vi "COP FSM.vi"   [LabVIEW 2009]
uses:
  COP Support Files/COP FSM States.ctl
  Support Files/JUDP Write Queue Element.ctl
  <vilib>/Platform/TimedLoop/XDataNode/XDataNode.xnode
  <vilib>/Platform/TimedLoop/XDataNode/loadlvalarms.vi
  <vilib>/Platform/TimedLoop/XDataNode/timing_clust.ctl
  <vilib>/Platform/TimedLoop/XDataNode/nitl_modes.ctl
  <vilib>/Platform/TimedLoop/XDataNode/wakeup.ctl
  <vilib>/Platform/TimedLoop/XDataNode/XDNodeRunTimeDep.lvlib
types:
  T1 = typedef "JUDP Write Queue Element.ctl" = cluster{"Encoded JAUS Message":string, "Destination ID":u32}
  T2 = typedef "COP FSM States.ctl" = enum16{"QueryStatus", "rQueryIdentification", "sReportIdentification", "sQueryServices", "rReportServices", "sQueryControl", "rReportControl", "sRequestControl", "rConfirmControl", "sResume", "sStandby", "sShutdown", "sQueryVelocityState", "sQueryLocalPose", "rSendWaypoints", "rExecuteWaypoints"}
  T3 = typedef "XDNodeRunTimeDep.lvlib/timing_clust.ctl" = cluster{"Expected End [f-1]":u64, "Actual End [f-1]":u64, "Finished Late? [f-1]":bool, "Expected End [i-1]":u64, "Actual End [i-1]":u64, "Finished Late? [i-1]":bool, "Expected Start [i]":u64, "Actual Start [i]":u64, "Expected Start [f]":u64, "Actual Start [f]":u64, "Source Name":string, "Structure Name":string, "Period":i64, "Deadline":i64, "Offset":i64, "Start":i64, "Priority":i32, "Timeout":i32, "Mode":T4, "Wakeup Reason":T5, "Error":errorcluster, "Source Type":string, "Secondary Source Type":string, "Global End Time":u64, "Global Start Time":u64, "Frame Duration":u64, "Iteration Duration":u64, "Assigned CPU":i32, "I/O Scan Engine Mode":u32}
  T4 = typedef "XDNodeRunTimeDep.lvlib/nitl_modes.ctl" = enum32{"No Change", "Process missed periods, maintain original phase", "Discard missed periods, maintain original phase", "Process missed periods, ignore original phase", "Discard missed periods, ignore original phase"}
  T5 = typedef "XDNodeRunTimeDep.lvlib/wakeup.ctl" = enum32{"Normal", "Aborted", "Asynchronous wakeup", "Timing source error", "Timed loop error", "Timeout"}
  T6 = typedef "Address.ctl" = cluster{"Subsystem Id":u16, "Node Id":u8, "Component Id":u8}
  T7 = typedef "RequestIDRec.ctl" = cluster{"RequestId":u8, "Element List":T8[]}
  T8 = typedef "ElementRec.ctl" = cluster{"ElementUID":u16, " PreviousUID":u16, " NextUID":u16, "LocalWaypointRec":T9}
  T9 = typedef "LocalWaypointRec.ctl" = cluster{"Presence Vector":u8, " X":dbl, " Y":dbl, " Z":dbl, "Roll":dbl, "Pitch":dbl, "Yaw":dbl, "Waypoint Tolerance":dbl, "Path Tolerance":dbl, "Is Active?":bool}
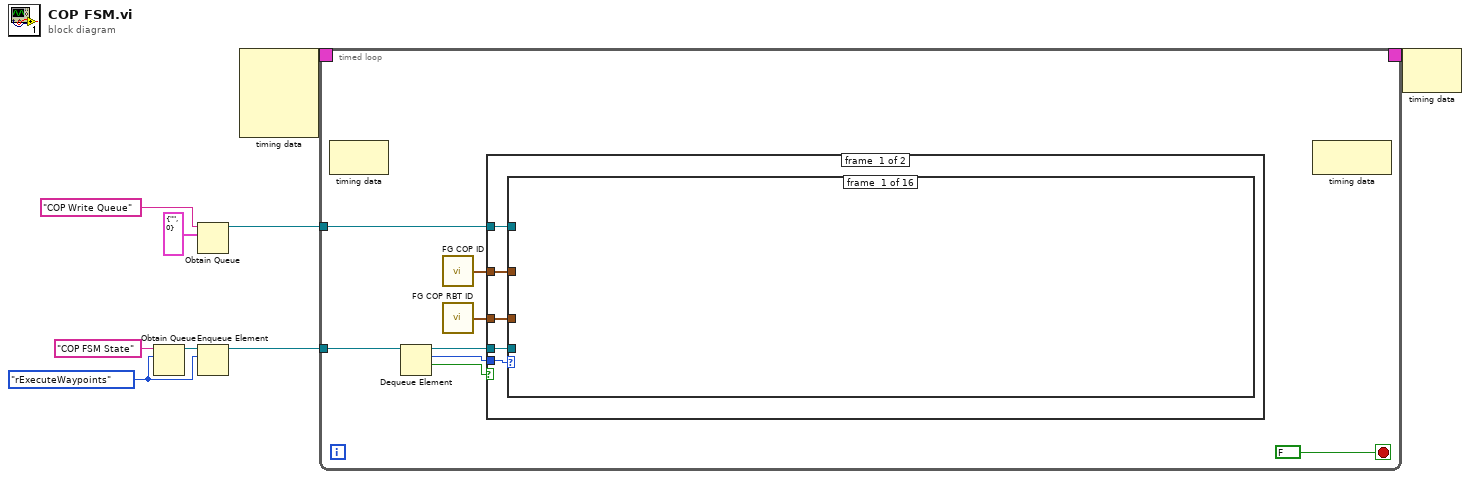
[diagram p0: block diagram]
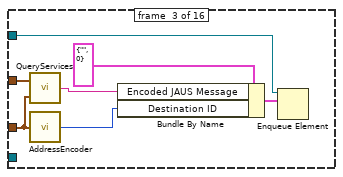
[diagram p3: hidden frame]
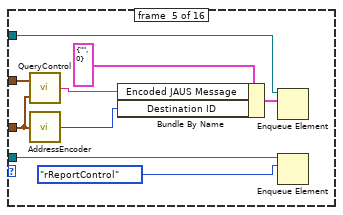
[diagram p5: hidden frame]
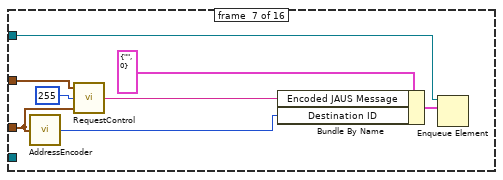
[diagram p7: hidden frame]
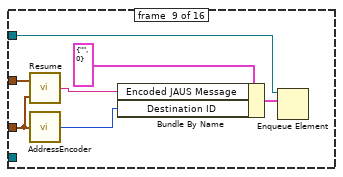
[diagram p9: hidden frame]
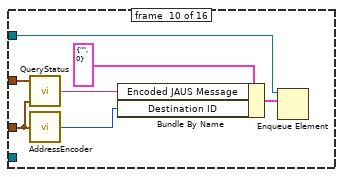
[diagram p10: hidden frame]
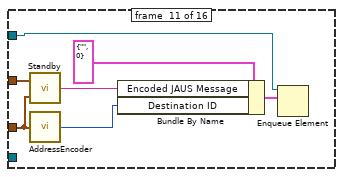
[diagram p11: hidden frame]
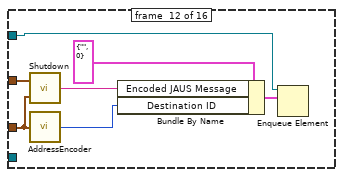
[diagram p12: hidden frame]
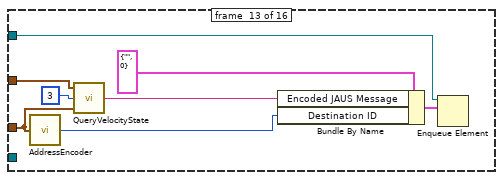
[diagram p13: hidden frame]
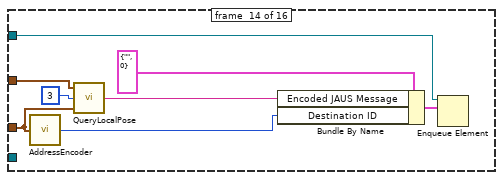
[diagram p14: hidden frame]
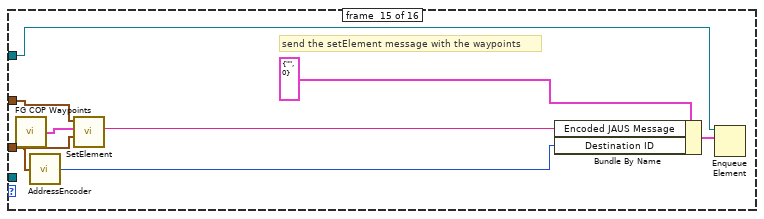
[diagram p15: hidden frame]
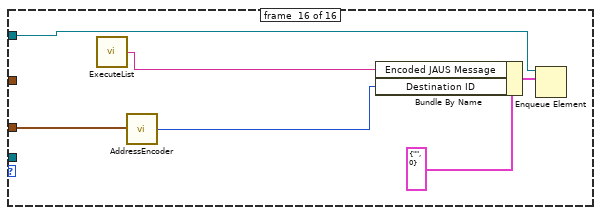
[diagram p16: hidden frame]
diagram:
  w6 = COP_FSM_States."rExecuteWaypoints" ("COP FSM States")
  n1 = Obtain Queue(name (unnamed)="COP FSM State", element data type=w6) -> (queue out=w8:refnum<queue>)  [unwired: 3 in, 2 out]
  n2 = Obtain Queue(name (unnamed)="COP Write Queue", element data type=T1 {"Encoded JAUS Message"="", "Destination ID"=0} ("Cluster")) -> (queue out=w3:refnum<queue>)  [unwired: 3 in, 2 out]
  n3 = Enqueue Element(queue=w8, element=w6) -> (queue out=w7:refnum<queue>)  [unwired: 2 in, 2 out]
  n4 = node-c288() -> (w2:T3)  [unwired: 4 in]
  n5 = timed-loop {
    tunnel: w7 -> [w17]
    tunnel: w3 -> [w14]
    timing: w2 -> [_]
    timing-out: [_] -> w1
    stop <- FALSE stop-if-true
    n6 = node-c288() -> ()  [unwired: 1 in, 1 out]
    n7 = Dequeue Element(queue=w17) -> (queue out=w15:refnum<queue>, element=w16:T2, timed out?=w10:bool)  [unwired: 2 in, 1 out]
    n8 = call "FG COP ID.vi"() -> ("COP ID out"=w13:T6)  [unwired: 2 in]
    n9 = call "FG COP RBT ID.vi"() -> ("RBT ID out"=w12:T6)  [unwired: 2 in]
    n10 = case shown="False" w10 {
      tunnel: w16 -> [w24 _]
      tunnel: w15 -> [w23 _]
      tunnel: w14 -> [w22 _]
      tunnel: w13 -> [w21 _]
      tunnel: w12 -> [w20 _]
      frame #0 {
        n11 = case shown="\"rExecuteWaypoints\"" w24 {
          tunnel: w23 -> [_ _ _ _ w39 _ _ _ _ _ _ _ _ _ _ _]
          tunnel: w22 -> [_ _ w27 _ w32 _ w46 _ w50 w62 w66 w73 w79 w85 w97 w103]
          tunnel: w21 -> [_ _ w31 _ w35 _ w48 _ w55 w57 w65 w72 w84 w91 w96 _]
          tunnel: w20 -> [_ _ w26 _ w36 _ w43 _ w51 w56 w63 w70 w78 w87 w95 w106]
          frame #0 {
          }
          frame #1 {
          }
          frame #2 {
            n12 = call "QueryServices.vi"("Destination"=w26, "Source"=w31) -> ("Encoded JAUS Message"=w25:string)
            n13 = call "AddressEncoder.vi"("Address Cluster"=w26) -> ("Address"=w28:u32)
            n14 = Bundle By Name(cluster=T1 {"Encoded JAUS Message"="", "Destination ID"=0} ("element"), "Encoded JAUS Message"=w25, "Destination ID"=w28) -> (w29:T1)
            n15 = Enqueue Element(queue=w27, element=w29) -> ()  [unwired: 2 in, 3 out]
          }
          frame #3 {
          }
          frame #4 {
            n16 = call "QueryControl.vi"("Destination"=w36, "Source"=w35) -> ("Encoded JAUS Message"=w37:string)
            n17 = call "AddressEncoder.vi"("Address Cluster"=w36) -> ("Address"=w34:u32)
            n18 = Bundle By Name(cluster=T1 {"Encoded JAUS Message"="", "Destination ID"=0} ("element"), "Encoded JAUS Message"=w37, "Destination ID"=w34) -> (w33:T1)
            n19 = Enqueue Element(queue=w32, element=w33) -> ()  [unwired: 2 in, 3 out]
            n20 = Enqueue Element(queue=w39, element=COP_FSM_States."rReportControl" ("COP FSM States")) -> ()  [unwired: 2 in, 3 out]
          }
          frame #5 {
          }
          frame #6 {
            n21 = call "AddressEncoder.vi"("Address Cluster"=w43) -> ("Address"=w44:u32)
            n22 = call "RequestControl.vi"("Destination"=w43, "AuthorityCode"=u8 255, "Source"=w48) -> ("Encoded JAUS Message"=w42:string)
            n23 = Bundle By Name(cluster=T1 {"Encoded JAUS Message"="", "Destination ID"=0} ("Cluster"), "Encoded JAUS Message"=w42, "Destination ID"=w44) -> (w41:T1)
            n24 = Enqueue Element(queue=w46, element=w41) -> ()  [unwired: 2 in, 3 out]
          }
          frame #7 {
          }
          frame #8 {
            n25 = call "Resume.vi"("Destination"=w51, "Source"=w55) -> ("Encoded JAUS Message"=w52:string)
            n26 = call "AddressEncoder.vi"("Address Cluster"=w51) -> ("Address"=w53:u32)
            n27 = Bundle By Name(cluster=T1 {"Encoded JAUS Message"="", "Destination ID"=0} ("Cluster"), "Encoded JAUS Message"=w52, "Destination ID"=w53) -> (w49:T1)
            n28 = Enqueue Element(queue=w50, element=w49) -> ()  [unwired: 2 in, 3 out]
          }
          frame #9 {
            n29 = call "QueryStatus.vi"("Destination"=w56, "Source"=w57) -> ("Encoded JAUS Message"=w59:string)  [unwired: 1 in]
            n30 = call "AddressEncoder.vi"("Address Cluster"=w56) -> ("Address"=w58:u32)
            n31 = Bundle By Name(cluster=T1 {"Encoded JAUS Message"="", "Destination ID"=0} ("element"), "Encoded JAUS Message"=w59, "Destination ID"=w58) -> (w60:T1)
            n32 = Enqueue Element(queue=w62, element=w60) -> ()  [unwired: 2 in, 3 out]
          }
          frame #10 {
            n33 = call "Standby.vi"("Destination"=w63, "Source"=w65) -> ("Encoded JAUS Message"=w64:string)
            n34 = call "AddressEncoder.vi"("Address Cluster"=w63) -> ("Address"=w68:u32)
            n35 = Bundle By Name(cluster=T1 {"Encoded JAUS Message"="", "Destination ID"=0} ("Cluster"), "Encoded JAUS Message"=w64, "Destination ID"=w68) -> (w67:T1)
            n36 = Enqueue Element(queue=w66, element=w67) -> ()  [unwired: 2 in, 3 out]
          }
          frame #11 {
            n37 = call "Shutdown.vi"("Destination"=w70, "Source"=w72) -> ("Encoded JAUS Message"=w71:string)
            n38 = call "AddressEncoder.vi"("Address Cluster"=w70) -> ("Address"=w76:u32)
            n39 = Bundle By Name(cluster=T1 {"Encoded JAUS Message"="", "Destination ID"=0} ("Cluster"), "Encoded JAUS Message"=w71, "Destination ID"=w76) -> (w74:T1)
            n40 = Enqueue Element(queue=w73, element=w74) -> ()  [unwired: 2 in, 3 out]
          }
          frame #12 {
            n41 = call "AddressEncoder.vi"("Address Cluster"=w78) -> ("Address"=w82:u32)
            n42 = call "QueryVelocityState.vi"("Destination"=w78, "PresenceVector"=u16 3, "Source"=w84) -> ("Encoded JAUS Message"=w77:string)
            n43 = Bundle By Name(cluster=T1 {"Encoded JAUS Message"="", "Destination ID"=0} ("Cluster"), "Encoded JAUS Message"=w77, "Destination ID"=w82) -> (w80:T1)
            n44 = Enqueue Element(queue=w79, element=w80) -> ()  [unwired: 2 in, 3 out]
          }
          frame #13 {
            n45 = call "AddressEncoder.vi"("Address Cluster"=w87) -> ("Address"=w90:u32)
            n46 = call "QueryLocalPose.vi"("Destination"=w87, "PresenceVector"=u16 3, "Source"=w91) -> ("Encoded JAUS Message"=w86:string)
            n47 = Bundle By Name(cluster=T1 {"Encoded JAUS Message"="", "Destination ID"=0} ("Cluster"), "Encoded JAUS Message"=w86, "Destination ID"=w90) -> (w88:T1)
            n48 = Enqueue Element(queue=w85, element=w88) -> ()  [unwired: 2 in, 3 out]
          }
          frame #14 {
            # "send the setElement message with the waypoints"
            n49 = call "FG COP Waypoints.vi"() -> ("COP Waypoints out"=w93:T7)  [unwired: 2 in]
            n50 = call "AddressEncoder.vi"("Address Cluster"=w95) -> ("Address"=w98:u32)
            n51 = call "SetElement.vi"("Destination"=w95, "RequestIDRec"=w93, "Source"=w96) -> ("Encoded JAUS Message"=w94:string)  [unwired: 8 in]
            n52 = Bundle By Name(cluster=T1 {"Encoded JAUS Message"="", "Destination ID"=0} ("Cluster"), "Encoded JAUS Message"=w94, "Destination ID"=w98) -> (w100:T1)
            n53 = Enqueue Element(queue=w97, element=w100) -> ()  [unwired: 2 in, 3 out]
          }
          frame #15 {
            n54 = call "ExecuteList.vi"() -> ("Encoded JAUS Message"=w104:string)  [unwired: 3 in]
            n55 = call "AddressEncoder.vi"("Address Cluster"=w106) -> ("Address"=w105:u32)
            n56 = Bundle By Name(cluster=T1 {"Encoded JAUS Message"="", "Destination ID"=0} ("Cluster"), "Encoded JAUS Message"=w104, "Destination ID"=w105) -> (w101:T1)
            n57 = Enqueue Element(queue=w103, element=w101) -> ()  [unwired: 2 in, 3 out]
          }
        }
      }
      frame #1 {
      }
    }
    n58 = node-c288() -> ()  [unwired: 1 in, 1 out]
  }
  n59 = node-c288(w1) -> ()  [unwired: 1 out]
